vi "Read Compiler.vi"(8 "error in (no error)":errorcluster, 11 "Python Protocol in":refnum<class "Python Protocol.lvclass">) -> (0 "error out":errorcluster, 2 "Compiler":refnum<vi>, 3 "Python Protocol out":refnum<class "Python Protocol.lvclass">)   [LabVIEW 2012, in "Python Protocol Actor.lvlib" / "Python Protocol.lvclass"]
uses:
  Python Protocol.lvclass
  Python Protocol.lvclass/Python Protocol.ctl
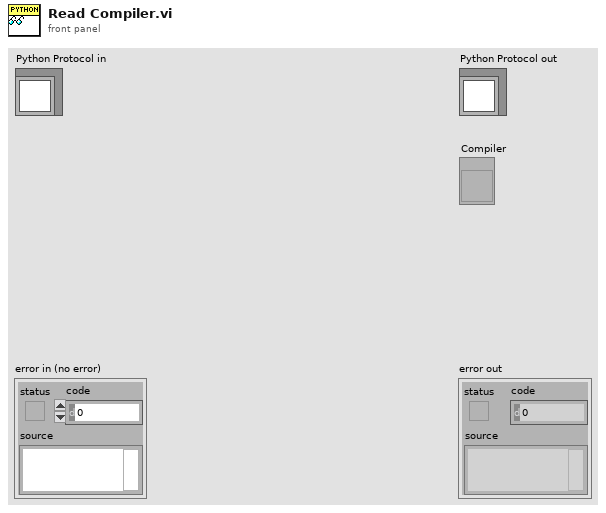
[diagram p1: front panel]
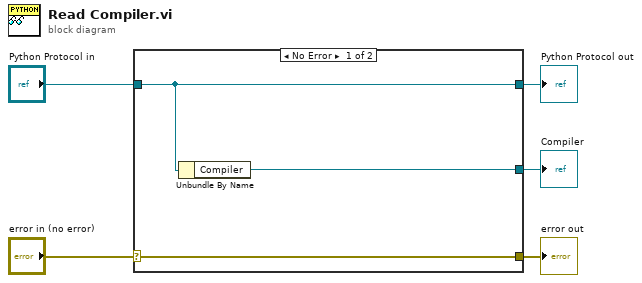
[diagram p0: block diagram]
diagram:
  n1 = case shown="No Error" "error in (no error)" {
    selector: "error in (no error)" -> [w8 w9]
    tunnel: [w8 w9] -> w4
    tunnel: [w7 w10] -> w2
    tunnel: "Python Protocol in" -> [w7 w10]
    tunnel: [w6 _] -> w1
    frame No Error {
      n2 = Unbundle By Name(w7) -> ("Compiler"=w6:refnum<vi>)
    }
    frame Error {
    }
  }
  "error out" <- w4
  "Python Protocol out" <- w2
  "Compiler" <- w1
